vi "SignalSenderLoop.SetSignalsFrame.vi"(8 "error in (no error)":errorcluster, 10 "SignalFrameSet":T1={"Port_No."="CAN1", "计数Count"=FALSE, "校验CheckSum"=FALSE, "MessageFrame"="ESP_1\nLRA110", "校验算法名称"=""}, 11 "SignalSenderLoop":refnum<class "SignalSenderLoop.lvclass">) -> (0 "error out":errorcluster, 3 "SignalSenderLoop out":refnum<class "SignalSenderLoop.lvclass">)   [LabVIEW 2020, in "ECU_Diagnose.lvlib" / "SignalSenderLoop.lvclass"]
doc: "---------------------------------------------------------------\nJKI State Machine Objects™\nhttp://jki.net/state-machine-objects/\nCopyright (C) 2005-2015, JKI <info@jki.net>\nALL RIGHTS RESERVEDJKI State Machine Objects (SMO) 1.0.0.5\nJKI - JKI\nCopyright (c) 2016, JKI"
uses:
  SignalSenderLoop.lvclass
  subvi/SignalFrameSet.ctl
  SignalSenderLoop.lvclass/SignalSenderLoop.ctl
panel:
  # "For instructions on how to use the JKI State Machine Objects, examples and video tutorials, visit:\nhttp://jki.net/state-machine-objects/\n\nJKI State Machine Objects™\nhttp://jki.net/state-machine-objects/\nCopyright (C) 2005-2015, JKI <info@jki.net>\nALL RIGHTS RESERVED"
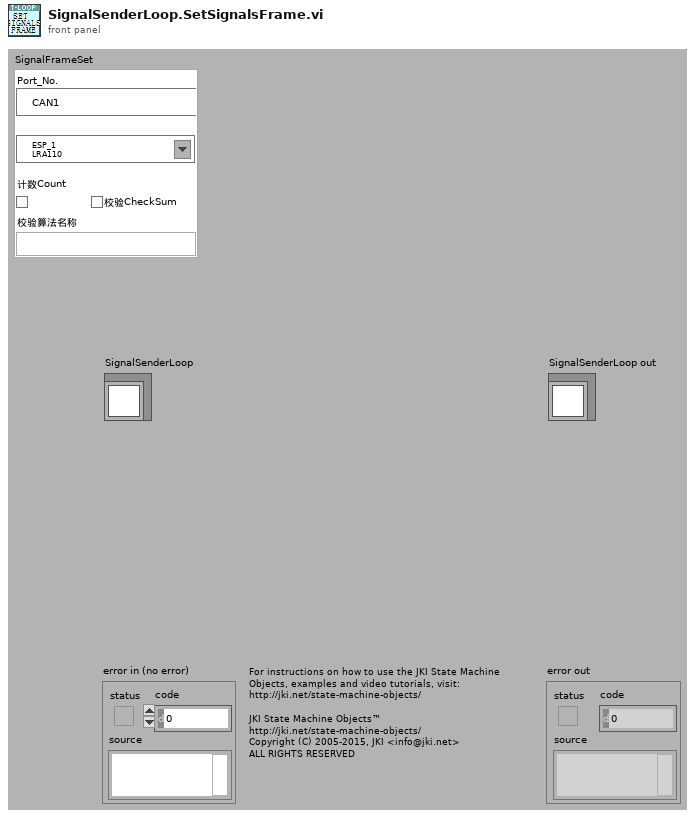
[diagram p1: front panel]
types:
  T1 = typedef "ECU_Diagnose.lvlib/SignalSenderLoop.lvclass/SignalFrameSet.ctl" = cluster{"Port_No.":refnum<k21>, "计数Count":bool, "校验CheckSum":bool, "MessageFrame":refnum<k21>, "校验算法名称":string}
  T2 = typedef "ECU_Diagnose.lvlib/SignalSenderLoop.lvclass/PrivateData--Ref.ctl" = refnum<data-value>
  T3 = typedef "ECU_Diagnose.lvlib/SignalSenderLoop.lvclass/PrivateData--Cluster.ctl" = cluster{"Public Events":T4, "Setpoint":T5, "Private Events":T6, "SignalFrameSet":T1}
  T4 = typedef "ECU_Diagnose.lvlib/SignalSenderLoop.lvclass/PublicEvents--Cluster.ctl" = cluster{"Setpoint Changed":refnum<user-event>, "Value Changed":refnum<user-event>}
  T5 = typedef "ECU_Diagnose.lvlib/SignalSenderLoop.lvclass/Data.ctl" = dbl
  T6 = typedef "ECU_Diagnose.lvlib/SignalSenderLoop.lvclass/PrivateEvents--Cluster.ctl" = cluster{"AsyncMethod":refnum<user-event>, "SignalCMDArry":refnum<user-event>}
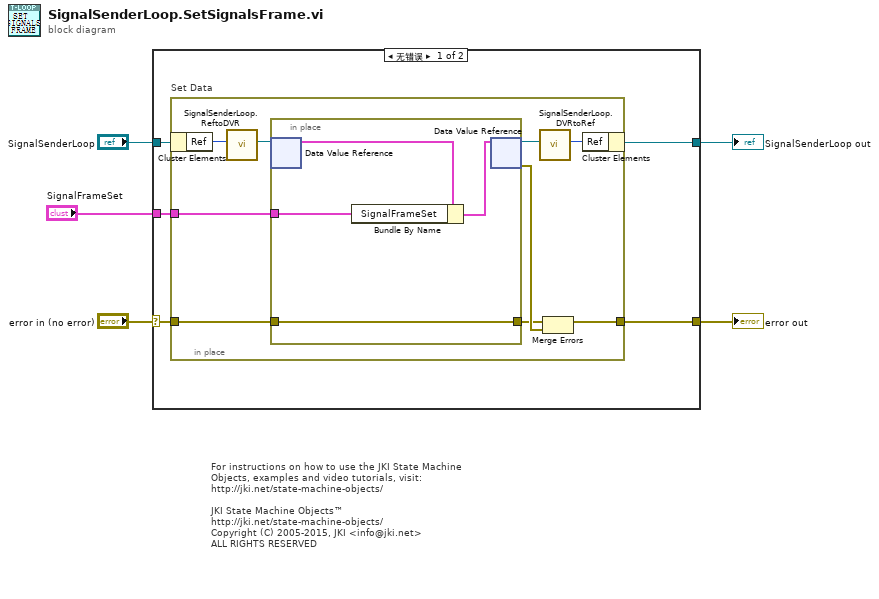
[diagram p0: block diagram]
diagram:
  # "For instructions on how to use the JKI State Machine Objects, examples and video tutorials, visit:\nhttp://jki.net/state-machine-objects/\n\nJKI State Machine Objects™\nhttp://jki.net/state-machine-objects/\nCopyright (C) 2005-2015, JKI <info@jki.net>\nALL RIGHTS RESERVED"
  n1 = case shown="无错误" "error in (no error)" {
    selector: "error in (no error)" -> [w9 w24]
    tunnel: "SignalSenderLoop" -> [w10 w25]
    tunnel: [w8 w24] -> w4
    tunnel: [w7 w25] -> w3
    tunnel: "SignalFrameSet" -> [w6 _]
    frame No Error {
      n2 = in-place "Set Data" {
        in-place-border: w9 -> [w19]
        in-place-border: [w16] -> w8
        in-place-border: w6 -> [w11]
        n3 = in-place-cluster #1(w10) -> ("Ref"=w15:u32)
        n4 = call "SignalSenderLoop.ReftoDVR.vi"("Ref"=w15) -> ("Ref"=w14:T2)  [unwired: 10 in]
        n5 = in-place {
          in-place-border: w19 -> [w23]
          in-place-border: [w23] -> w17
          in-place-border: w11 -> [w20]
          n6 = in-place-dvr #2(w14) -> (w22:T3)  [unwired: 1 out]
          n7 = Bundle By Name(cluster=w22, "SignalFrameSet"=w20) -> (w21:T3)
          n8 = in-place-dvr #2(w21) -> (w13:T2, w18:errorcluster)
        }
        n9 = call "SignalSenderLoop.DVRtoRef.vi"("Ref"=w13) -> ("Ref"=w12:u32)  [unwired: 10 in]
        n10 = Merge Errors(w17, w18) -> (w16:errorcluster)
        n11 = in-place-cluster #1("Ref"=w12) -> (w7:refnum<class "SignalSenderLoop.lvclass">)
      }
    }
    frame Error {
    }
  }
  "error out" <- w4
  "SignalSenderLoop out" <- w3
